vi "temp.vi"() -> (0 "number 2":dbl, 1 "Chaîne":string)   [LabVIEW 2018]
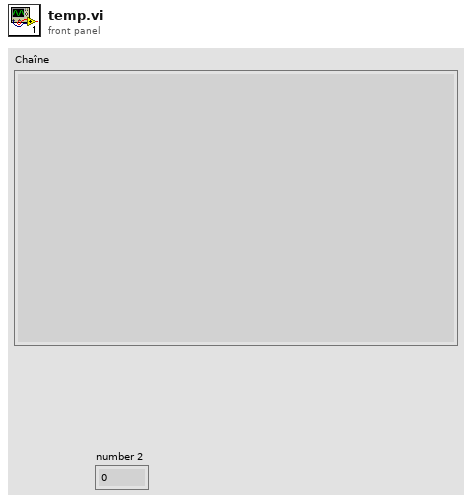
[diagram p1: front panel]
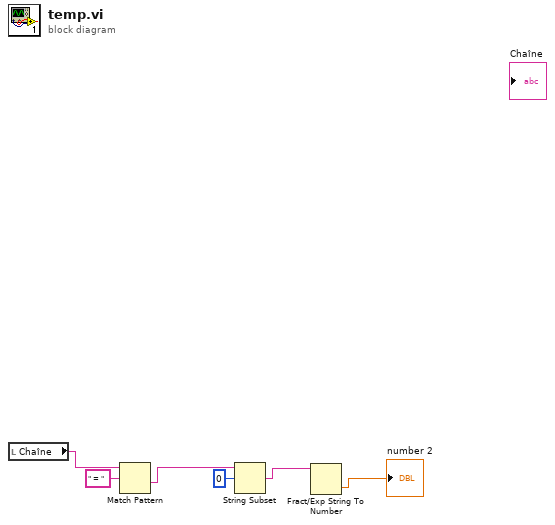
[diagram p0: block diagram]
diagram:
  n1 = local read "Chaîne"() -> (w6:string)
  n2 = Match Pattern(string=w6, regular expression=" = ") -> (after substring=w4:string)  [unwired: 1 in, 3 out]
  n3 = String Subset(string=w4, offset (0)=0) -> (substring=w2:string)  [unwired: 1 in]
  n4 = Fract/Exp String To Number(string=w2) -> (number=→"number 2":dbl)  [unwired: 3 in, 1 out]
